vi "CheckNumberOfLocalsRuleConstants.vi"() -> ()   [LabVIEW 2011]
panel:
  in  "Rule Setting Name":string="Maximum Number of Locals"
  in  "Rule Id":string="NI_CheckNumberOfLocalsLVExample"
  # "Constants used by the CheckNumberOfLocals analysis module"
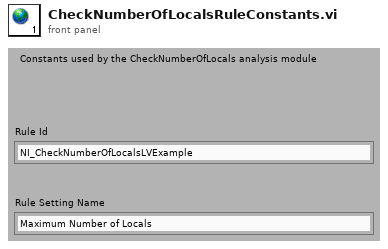
[diagram p1: front panel]
diagram:
